vi "FindSimilarDataFrom2DArray.vi"(9 "column index":u16, 10 "search string":string, 11 "array in":string[][](array[string])) -> (2 "is empty?":bool, 3 "array out":string[][](array[string]))   [LabVIEW 2018, in "Library-Ctrl.lvlib"]
uses:
  Library-Ctrl.lvlib
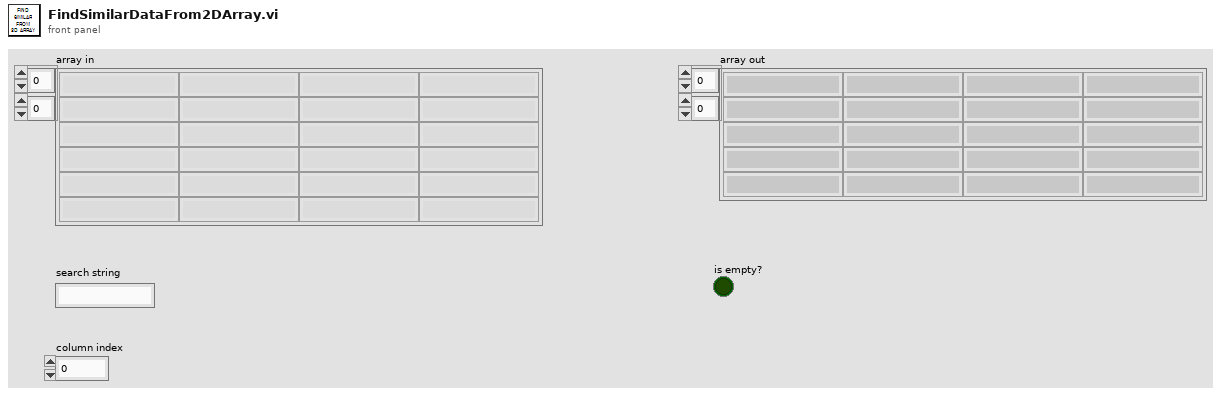
[diagram p1: front panel]
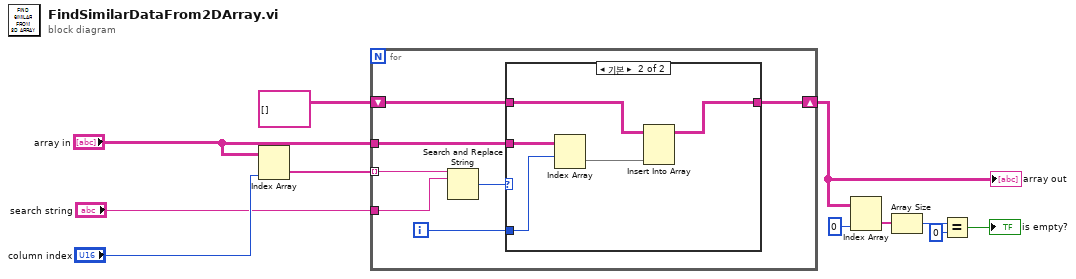
[diagram p0: block diagram]
diagram:
  n1 = Index Array(array="array in", index (col)="column index") -> (element=w2:string[])  [unwired: 1 in]
  n2 = for {
    tunnel: "search string" -> [w14]
    shift-right: [w17] -> w8
    shift-left: string[][] [] ("result") -> [w18]
    tunnel: "array in" -> [w16]
    tunnel: w2 -> [w15] mode=indexing
    i -> [w12]
    n3 = Search and Replace String(input string=w15, search string=w14) -> (number of replacements=w13:i32)  [unwired: 6 in, 3 out]
    n4 = case shown="기본" w13 {
      tunnel: w18 -> [w19 w24]
      tunnel: [w19 w23] -> w17
      tunnel: w16 -> [_ w22]
      tunnel: w12 -> [_ w20]
      frame 0 {
      }
      frame Default {
        n5 = Index Array(array=w22, index (row)=w20) -> (element=w21:string[])  [unwired: 1 in]
        n6 = Insert Into Array(array=w24, new element=w21) -> (w23:string[][])  [unwired: 2 in]
      }
    }
  }
  "array out" <- w8
  n7 = Index Array(array=w8, index (col)=0 ("비활성화된 인덱스 (열)")) -> (element=w6:string[])  [unwired: 1 in]
  n8 = Array Size(array=w6) -> (size(s)=w5:i32)
  n9 = Equal?(x=w5, y=0) -> (x = y?=→"is empty?":bool)
